vi "Module.Destructor.vi"(8 "error in":errorcluster, 11 "Sys":T1) -> (0 "error out":errorcluster)   [LabVIEW 2024, in "EQMF.lvlib" / "Module Utils.lvlib"]
uses:
  Module Utils.lvlib
  Module Sys Info.ctl
  Config/Stored Controls/Class.SaveCtrls.lvclass
  Event Log/Event Notification/Event Notification.lvclass
  Config/App Data/Class.AppData.lvclass
  Subscription/Subscription.lvclass
  Queues/Q.Element.ctl
  Module.SW Version Info.ctl
  Module Config.ctl
  Module.Working Dirs.ctl
  Queues/Queue Utils.lvlib
  Controls/Controls.lvlib
panel:
  # "Name, PN, Version, Note"
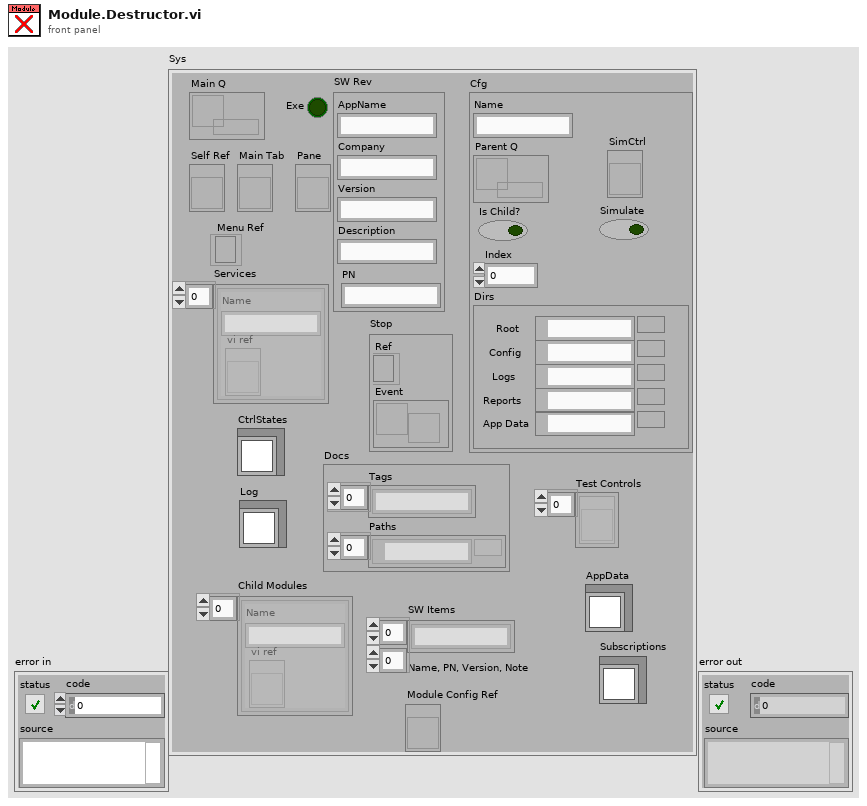
[diagram p1: front panel]
types:
  T1 = typedef "EQMF.lvlib/Module Utils.lvlib/Module Sys Info.ctl" = cluster{"Main Q":refnum<queue>, "Exe":bool, "SW Rev":T2, "Self Ref":refnum<vi>, "Main Tab":refnum<vi>, "Pane":refnum<vi>, "Stop":cluster{"Ref":refnum<event-registration>, "Event":refnum<user-event>}, "Cfg":T3, "Services":cluster{"Name":string, "vi ref":refnum<vi>}[], "Menu Ref":refnum<k9>, "CtrlStates":refnum<class "Class.SaveCtrls.lvclass">, "Docs":cluster{"Tags":string[], "Paths":path[]}, "Log":refnum<class "Event Notification.lvclass">, "Test Controls":refnum<vi>[], "Child Modules":cluster{"Name":string, "vi ref":refnum<vi>}[], "SW Items":string[][], "AppData":refnum<class "Class.AppData.lvclass">, "Subscriptions":refnum<class "Subscription.lvclass">, "Module Config Ref":refnum<vi>}
  T2 = typedef "EQMF.lvlib/Module Utils.lvlib/Module.SW Version Info.ctl" = cluster{"AppName":string, "Company":string, "Version":string, "Description":string, "PN":string}
  T3 = typedef "EQMF.lvlib/Module Utils.lvlib/Module Config.ctl" = cluster{"Name":string, "Parent Q":refnum<queue>, "Is Child?":bool, "Index":i32, "Dirs":T4, "Simulate":bool, "SimCtrl":refnum<vi>}
  T4 = typedef "EQMF.lvlib/Module Utils.lvlib/Module.Working Dirs.ctl" = cluster{"Root":path, "Config":path, "Logs":path, "Reports":path, "App Data":path}
  T5 = typedef "KATE_Lib.lvlib/Module Utils.lvlib/Module Config.ctl" = cluster{"Name":string, "Parent Q":refnum<queue>, "Is Child?":bool, "Index":i32, "Dirs":T6, "Simulate":bool, "SimCtrl":refnum<vi>}
  T6 = typedef "KATE_Lib.lvlib/Module Utils.lvlib/Module.Working Dirs.ctl" = cluster{"Root":path, "Config":path, "Logs":path, "Reports":path, "App Data":path}
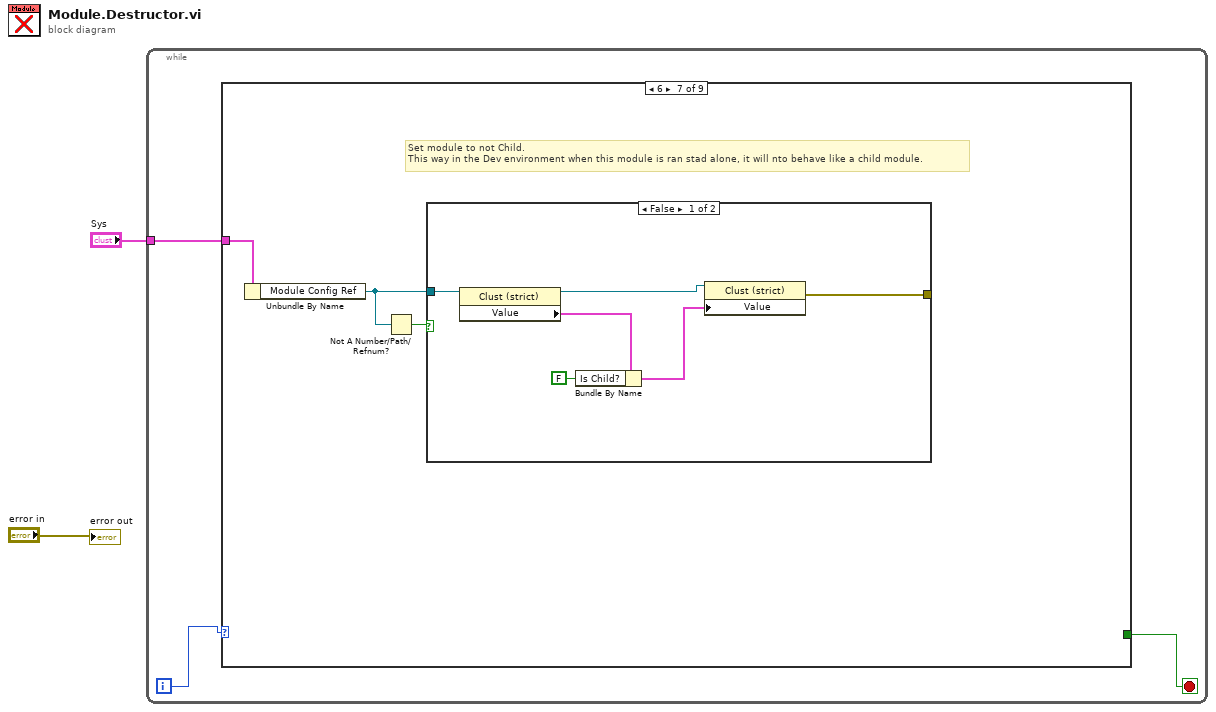
[diagram p0: block diagram]
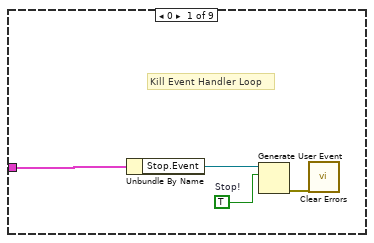
[diagram p2: hidden frame]
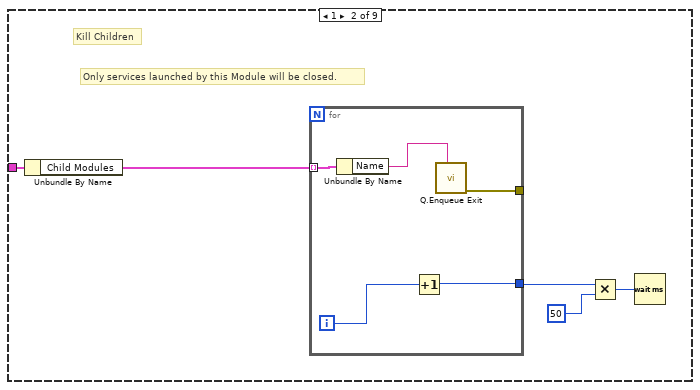
[diagram p3: hidden frame]
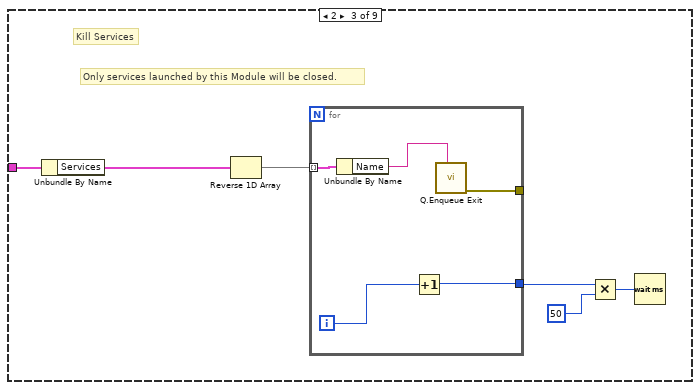
[diagram p4: hidden frame]
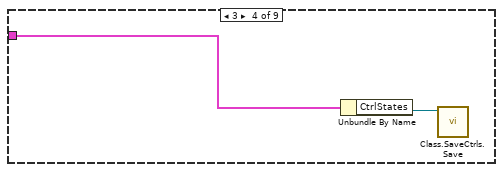
[diagram p5: hidden frame]
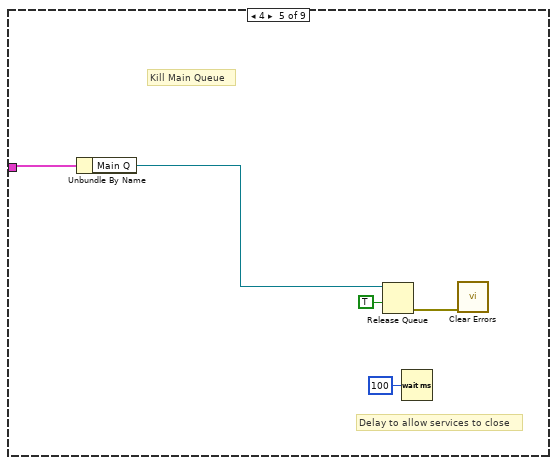
[diagram p6: hidden frame]
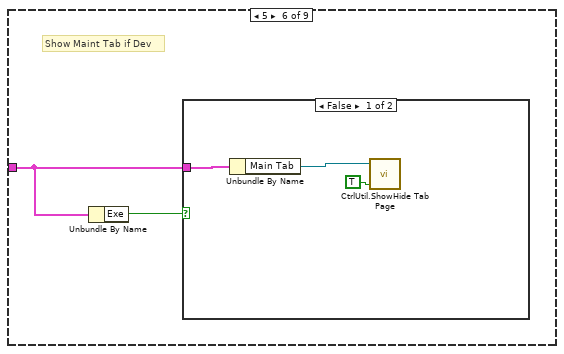
[diagram p7: hidden frame]
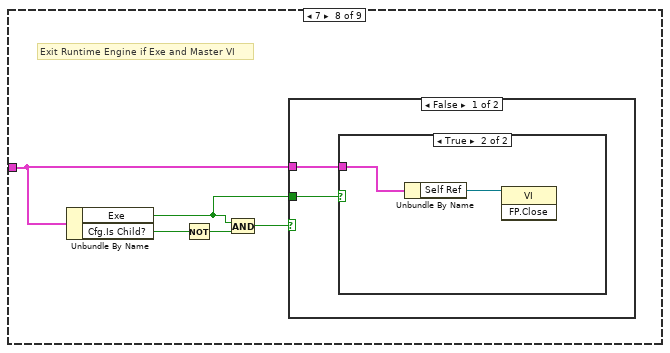
[diagram p10: hidden frame]
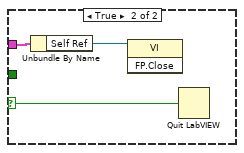
[diagram p12: hidden frame]
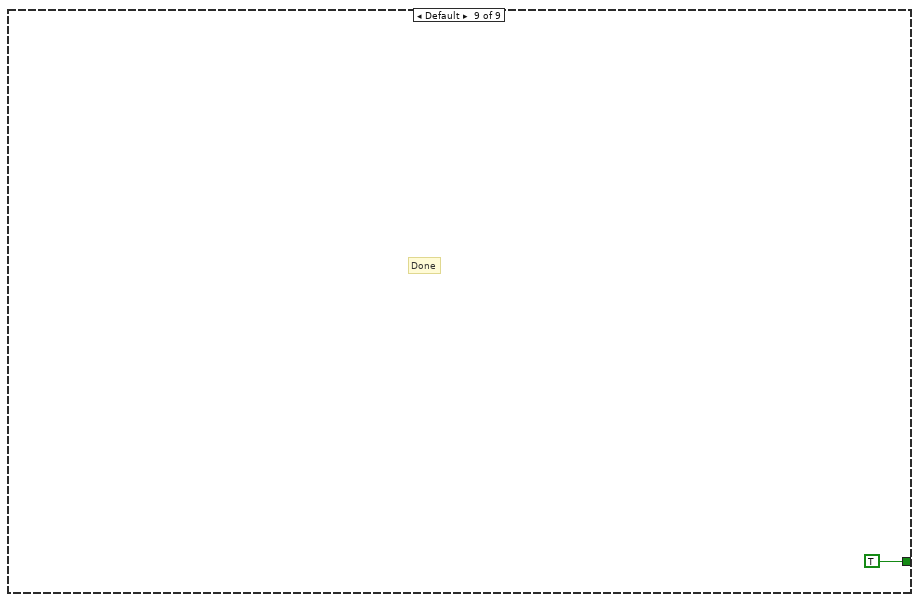
[diagram p13: hidden frame]
diagram:
  n1 = while {
    tunnel: "Sys" -> [w4]
    i -> [w5]
    stop <- w3 stop-if-true
    n2 = case shown="6" w5 {
      tunnel: [_ _ _ _ _ _ _ _ TRUE] -> w3
      tunnel: w4 -> [w9 w14 w25 w31 w36 w39 w45 w56 _]
      frame 0 {
        w7 = TRUE  # Stop!
        # "Kill Event Handler Loop"
        n3 = Unbundle By Name(w9) -> ("Stop.Event"=w8:refnum<user-event>)
        n4 = Generate User Event(user event=w8, event data cluster=w7) -> (error out=w6:errorcluster)  [unwired: 2 in, 1 out]
        n5 = call <vilib>:"Clear Errors.vi"("error in (no error)"=w6) -> ()  [unwired: 5 in, 2 out]
      }
      frame 1 {
        # "Only services launched by this Module will be closed."
        # "Kill Children"
        n6 = Unbundle By Name(w14) -> ("Child Modules"=w10:cluster{"Name":string, "vi ref":refnum<vi>}[])
        n7 = for {
          tunnel: w10 -> [w19] mode=indexing
          tunnel: [w18] -> _
          tunnel: [w16] -> w11
          i -> [w17]
          n8 = Unbundle By Name(w19) -> ("Name"=w15:string)
          n9 = Increment(x=w17) -> (x+1=w16:i32)
          n10 = call "Q.Enqueue Exit.vi"("Q Name"=w15) -> ("error out"=w18:errorcluster)  [unwired: 9 in, 1 out]
        }
        n11 = Multiply(x=w11, y=u32 50 ("milliseconds to wait")) -> (x*y=w12:u32)
        n12 = Wait (ms)(milliseconds to wait=w12) -> ()  [unwired: 1 out]
      }
      frame 2 {
        # "Only services launched by this Module will be closed."
        # "Kill Services"
        n13 = Unbundle By Name(w25) -> ("Services"=w24:cluster{"Name":string, "vi ref":refnum<vi>}[])
        n14 = Reverse 1D Array(array=w24) -> (reversed array=w23:cluster{"Name":string, "vi ref":refnum<vi>}[])
        n15 = for {
          tunnel: w23 -> [w30] mode=indexing
          tunnel: [w29] -> _
          tunnel: [w27] -> w20
          i -> [w28]
          n16 = Unbundle By Name(w30) -> ("Name"=w26:string)
          n17 = Increment(x=w28) -> (x+1=w27:i32)
          n18 = call "Q.Enqueue Exit.vi"("Q Name"=w26) -> ("error out"=w29:errorcluster)  [unwired: 9 in, 1 out]
        }
        n19 = Multiply(x=w20, y=u32 50 ("milliseconds to wait")) -> (x*y=w21:u32)
        n20 = Wait (ms)(milliseconds to wait=w21) -> ()  [unwired: 1 out]
      }
      frame 3 {
        n21 = Unbundle By Name(w31) -> ("CtrlStates"=w32:refnum<class "Class.SaveCtrls.lvclass">)
        n22 = call-dynamic "Class.SaveCtrls.Save.vi"("CtrlStates In"=w32) -> ()  [unwired: 9 in, 2 out]
      }
      frame 4 {
        # "Delay to allow services to close"
        # "Kill Main Queue"
        n23 = Unbundle By Name(w36) -> ("Main Q"=w35:refnum<queue>)
        n24 = Release Queue(queue=w35, force destroy? (F)=TRUE) -> (error out=w33:errorcluster)  [unwired: 1 in, 2 out]
        n25 = Wait (ms)(milliseconds to wait=u32 100) -> ()  [unwired: 1 out]
        n26 = call <vilib>:"Clear Errors.vi"("error in (no error)"=w33) -> ()  [unwired: 5 in, 2 out]
      }
      frame 5 {
        # "Show Maint Tab if Dev"
        n27 = Unbundle By Name(w39) -> ("Exe"=w38:bool)
        n28 = case shown="False" w38 {
          tunnel: w39 -> [w40 _]
          frame False {
            n29 = Unbundle By Name(w40) -> ("Main Tab"=w42:refnum<vi>)
            n30 = call "CtrlUtil.ShowHide Tab Page.vi"("Show"=TRUE, "Tab Control"=w42) -> ()  [unwired: 3 in]
          }
          frame True {
          }
        }
      }
      frame 6 {
        # "Set module to not Child.\nThis way in the Dev environment when this module is ran stad alone, it will nto behave like a child module."
        n31 = Unbundle By Name(w45) -> ("Module Config Ref"=w43:refnum<vi>)
        n32 = Not A Number/Path/Refnum?(number/path/refnum=w43) -> (NaN/Path/Refnum?=w44:bool)
        n33 = case shown="False" w44 {
          tunnel: w43 -> [w51 _]
          tunnel: [w46 _] -> _
          frame False {
            n34 = property class="Clust (strict)"(reference=w51) -> (reference out=w49:refnum<vi>, "Value"=w50:T5)  [unwired: 1 in, 1 out]
            n35 = Bundle By Name(cluster=w50, "Is Child?"=FALSE) -> (w48:T5)
            n36 = property class="Clust (strict)"(reference=w49, "Value"=w48) -> (error out=w46:errorcluster)  [unwired: 1 in, 1 out]
          }
          frame True {
          }
        }
      }
      frame 7 {
        # "Exit Runtime Engine if Exe and Master VI"
        n37 = Unbundle By Name(w56) -> ("Exe"=w52:bool, "Cfg.Is Child?"=w54:bool)
        n38 = Not(x=w54) -> (.not. x?=w55:bool)
        n39 = And(x=w52, y=w55) -> (x .and. y?=w53:bool)
        n40 = case shown="False" w53 {
          selector: w53 -> [_ w63]
          tunnel: w56 -> [w57 w62]
          tunnel: w52 -> [w58 _]
          frame False {
            n41 = case shown="True" w58 {
              tunnel: w57 -> [_ w59]
              frame False {
              }
              frame True {
                n42 = Unbundle By Name(w59) -> ("Self Ref"=w60:refnum<vi>)
                n43 = invoke class="VI" method="FP.Close"(reference=w60) -> ()  [unwired: 2 in, 3 out]
              }
            }
          }
          frame True {
            n44 = Unbundle By Name(w62) -> ("Self Ref"=w61:refnum<vi>)
            n45 = invoke class="VI" method="FP.Close"(reference=w61) -> ()  [unwired: 2 in, 3 out]
            n46 = Quit LabVIEW(quit? (T)=w63) -> ()
          }
        }
      }
      frame Default {
        # "Done"
      }
    }
  }
  "error out" <- "error in"
